vi "LB_ItemIndex.vi"(11 "error in (no error)":errorcluster) -> (15 "error out":errorcluster)   [LabVIEW 2016, in "DronaTest.lvlib"]
uses:
  DronaTest.lvlib
  APIs/Stimulus/ControlValue/SetValueAuto.vi
  APIs/Stimulus/ControlValue/Controls/Listbox/SetValueByItemIndex.vi
  APIs/Assert/AssertControlValue/Equal.vi
  <vilib>/addons/_JKI Toolkits/Caraya/classes/Assert/Assert Error.vi
  APIs/Stimulus/VI/CloseVI.vi
  <vilib>/addons/_JKI Toolkits/Caraya/classes/Test/Test.lvclass
  Drona.lvlib
  <vilib>/SLL Toolkit/SLL Debug/SLL Debug.lvlib
  APIs/Stimulus/ControlValue/Controls/Listbox/StimulusListbox.lvlib
  APIs/Assert/AssertControlValue/AssertControlValue.lvlib
  APIs/Stimulus/ControlValue/ControlValue.lvlib
  <vilib>/addons/_JKI Toolkits/Caraya/classes/Assert/Assert.lvclass
  APIs/Stimulus/VI/VI.lvlib
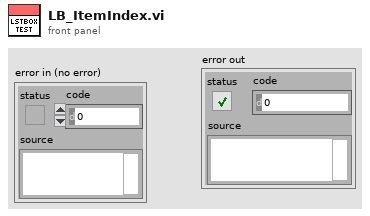
[diagram p1: front panel]
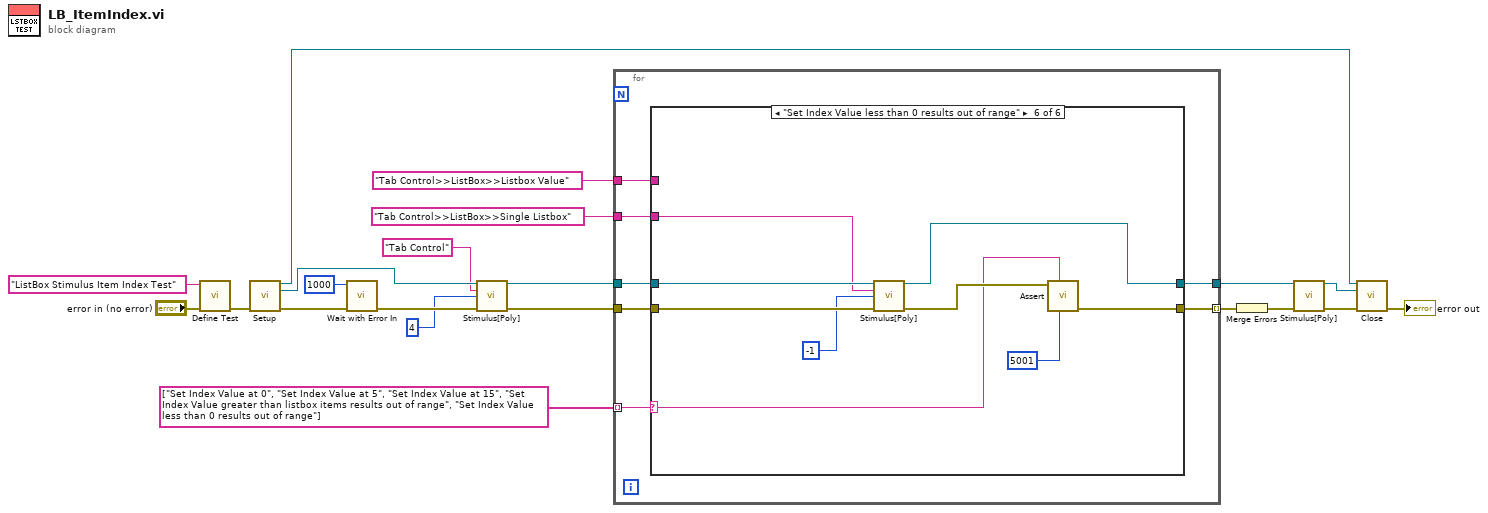
[diagram p0: block diagram]
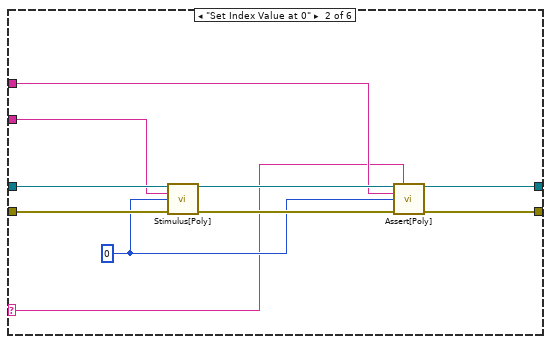
[diagram p3: hidden frame]
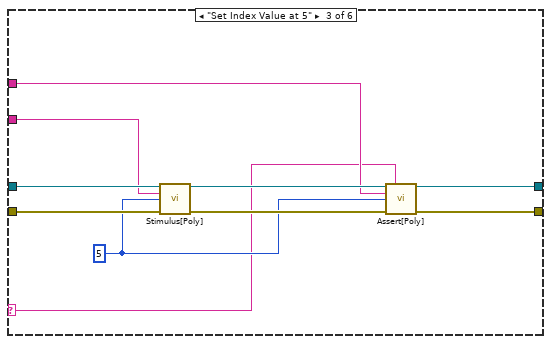
[diagram p4: hidden frame]
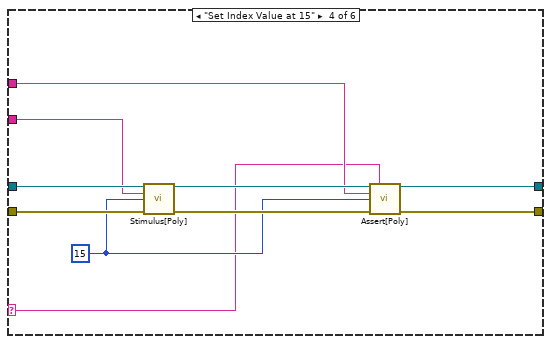
[diagram p5: hidden frame]
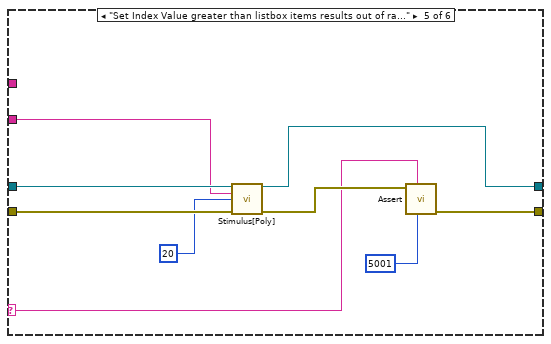
[diagram p6: hidden frame]
diagram:
  n1 = call <vilib>:"Define Test.vi"("error in (no error)"="error in (no error)", "Label (VI Title)"="ListBox Stimulus Item Index Test") -> ("error out"=w20:errorcluster)  [unwired: 9 in]
  n2 = call "Setup.vi"("error in"=w20) -> ("Application Ref"=w7:refnum<vi>, "VI Reference Out"=w14:refnum<vi>, "error out"=w19:errorcluster)  [unwired: 12 in]
  n3 = call <vilib>:"Wait with Error In.vi"("error in (no error)"=w19, "milliseconds to wait"=u32 1000) -> ("error out"=w16:errorcluster)  [unwired: 9 in]
  n4 = call-poly "Stimulus[Poly].vi"("VI Reference In"=w14, "Control Path"="Tab Control", "Value (Signaling)"=4, "error in"=w16) -> ("VI Reference Out"=w10:refnum<vi>, "error out"=w15:errorcluster)  [unwired: 10 in]
  n5 = for {
    tunnel: w10 -> [w27]
    tunnel: "Tab Control>>ListBox>>Single Listbox" ("Control Path") -> [w26]
    tunnel: "Tab Control>>ListBox>>Listbox Value" ("Control Path") -> [w25]
    tunnel: string[] ["Set Index Value at 0", "Set Index Value at 5", "Set Index Value at 15", "Set Index Value greater than listbox items results out of range", "Set Index Value less than 0 results out of range"] -> [w23] mode=indexing
    tunnel: [w22] -> w3
    tunnel: w15 -> [w28]
    tunnel: [w24] -> w2 mode=indexing
    n6 = case shown="\"Set Index Value less than 0 results out of range\"" w23 {
      selector: w23 -> [_ w31 w41 w51 w63 w72]
      tunnel: w28 -> [w30 w40 w50 w60 w69 w78]
      tunnel: w27 -> [w29 w39 w49 w59 w68 w77]
      tunnel: w26 -> [_ w35 w45 w55 w66 w75]
      tunnel: w25 -> [_ w34 w44 w54 _ _]
      tunnel: [w30 w33 w43 w53 w64 w73] -> w24
      tunnel: [w29 w32 w42 w52 w61 w70] -> w22
      frame Default {
      }
      frame "Set Index Value at 0" {
        w36 = 0 ("Item Index")
        n7 = call-poly "Stimulus[Poly].vi"("VI Reference In"=w39, "Control Path"=w35, "Item Index"=w36, "Error In"=w40) -> ("VI Reference Out"=w37:refnum<vi>, "Error Out"=w38:errorcluster)  [unwired: 10 in]
        n8 = call-poly "Assert[Poly].vi"("VI Reference In"=w37, "Test Label"=w31, "Control Path"=w34, "Control Value"=w36, "Error In"=w38) -> ("VI Reference Out"=w32:refnum<vi>, "Error Out"=w33:errorcluster)  [unwired: 8 in, 1 out]
      }
      frame "Set Index Value at 5" {
        w46 = 5 ("Item Index")
        n9 = call-poly "Stimulus[Poly].vi"("VI Reference In"=w49, "Control Path"=w45, "Item Index"=w46, "Error In"=w50) -> ("VI Reference Out"=w47:refnum<vi>, "Error Out"=w48:errorcluster)  [unwired: 10 in]
        n10 = call-poly "Assert[Poly].vi"("VI Reference In"=w47, "Test Label"=w41, "Control Path"=w44, "Control Value"=w46, "Error In"=w48) -> ("VI Reference Out"=w42:refnum<vi>, "Error Out"=w43:errorcluster)  [unwired: 8 in, 1 out]
      }
      frame "Set Index Value at 15" {
        w56 = 15 ("Item Index")
        n11 = call-poly "Stimulus[Poly].vi"("VI Reference In"=w59, "Control Path"=w55, "Item Index"=w56, "Error In"=w60) -> ("VI Reference Out"=w57:refnum<vi>, "Error Out"=w58:errorcluster)  [unwired: 10 in]
        n12 = call-poly "Assert[Poly].vi"("VI Reference In"=w57, "Test Label"=w51, "Control Path"=w54, "Control Value"=w56, "Error In"=w58) -> ("VI Reference Out"=w52:refnum<vi>, "Error Out"=w53:errorcluster)  [unwired: 8 in, 1 out]
      }
      frame "Set Index Value greater than listbox items results out of range" {
        n13 = call-poly "Stimulus[Poly].vi"("VI Reference In"=w68, "Control Path"=w66, "Item Index"=20, "Error In"=w69) -> ("VI Reference Out"=w61:refnum<vi>, "Error Out"=w65:errorcluster)  [unwired: 10 in]
        n14 = call-poly <vilib>:"Assert.vi"("error code (1)"=5001, "Label"=w63, "Error?"=w65) -> ("error out"=w64:errorcluster)  [unwired: 8 in]
      }
      frame "Set Index Value less than 0 results out of range" {
        n15 = call-poly "Stimulus[Poly].vi"("VI Reference In"=w77, "Control Path"=w75, "Item Index"=-1, "Error In"=w78) -> ("VI Reference Out"=w70:refnum<vi>, "Error Out"=w74:errorcluster)  [unwired: 10 in]
        n16 = call-poly <vilib>:"Assert.vi"("error code (1)"=5001, "Label"=w72, "Error?"=w74) -> ("error out"=w73:errorcluster)  [unwired: 8 in]
      }
    }
  }
  n17 = Merge Errors(w2) -> (w1:errorcluster)
  n18 = call-poly "Stimulus[Poly].vi"("VI Reference In"=w3, "error in"=w1) -> ("VI Reference Out"=w9:refnum<vi>, "error out"=w8:errorcluster)  [unwired: 12 in]
  n19 = call "Close.vi"("Application Ref"=w7, "VI Reference"=w9, "error in"=w8) -> ("error out"=→"error out":errorcluster)  [unwired: 12 in]
